vi "DRIVE_TURN.vi"(10 "argv":string[](array[string]), 11 "args":u8) -> ()   [LabVIEW 2011]
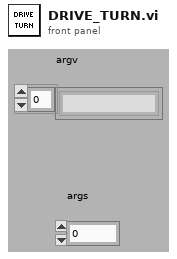
[diagram p1: front panel]
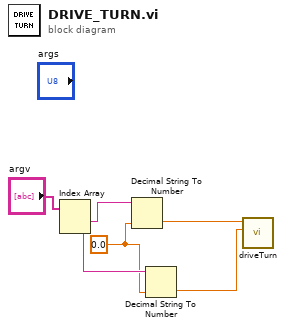
[diagram p0: block diagram]
diagram:
  w2 = 0.0
  n1 = Index Array(array="argv") -> (element #1=w5:string, element #2=w3:string)  [unwired: 2 in]
  n2 = Decimal String To Number(string=w5, default (0L)=w2) -> (number=w4:dbl)  [unwired: 1 in, 1 out]
  n3 = Decimal String To Number(string=w3, default (0L)=w2) -> (number=w1:dbl)  [unwired: 1 in, 1 out]
  n4 = call "driveTurn.vi"("fwd direction"=w1, "hdg target"=w4) -> ()  [unwired: 10 in]
